vi "modifyDatabasePath.vi"(5 "Database Path In":path) -> (2 "Database Path Out":path)   [LabVIEW 2019, in "Base de Datos.lvclass"]
doc: "This VI is modifying the database path if executed during runtime."
uses:
  Base de Datos.lvclass
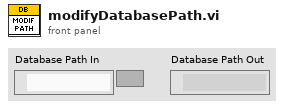
[diagram p1: front panel]
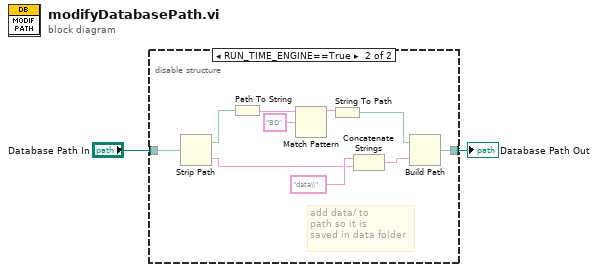
[diagram p0: block diagram]
diagram:
  n1 = disable-structure shown="RUN_TIME_ENGINE==True" {
    disable-tunnel: "Database Path In" -> [w3 w13]
    disable-tunnel: [w3 w12] -> w1
    frame condition #0 (active) {
      # "Do nothing"
    }
    frame condition #1 {
      # "add data/ to \npath so it is \nsaved in data folder"
      n2 = Strip Path(path=w13) -> (stripped path=w5:path, name=w9:string)
      n3 = Path To String(path=w5) -> (string=w8:string)
      n4 = Match Pattern(string=w8, regular expression="BD") -> (before substring=w6:string)  [unwired: 1 in, 3 out]
      n5 = String To Path(string=w6) -> (path=w4:path)
      n6 = Concatenate Strings("data\\" ("string"), w9) -> (w11:string)
      n7 = Build Path(base path=w4, name or relative path=w11) -> (appended path=w12:path)
    }
  }
  "Database Path Out" <- w1
